vi "Array for Graph Sub VI.vi"(10 "Array in":dbl[][](array[numeric]), 11 "data":dbl[](array[numeric])) -> (2 "Cluster":cluster{dbl[], dbl[]}, 3 "Array out":dbl[][](array[numeric]))   [LabVIEW 2011]
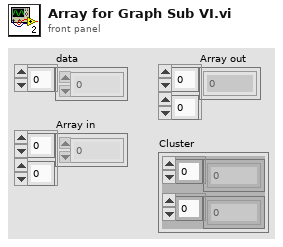
[diagram p1: front panel]
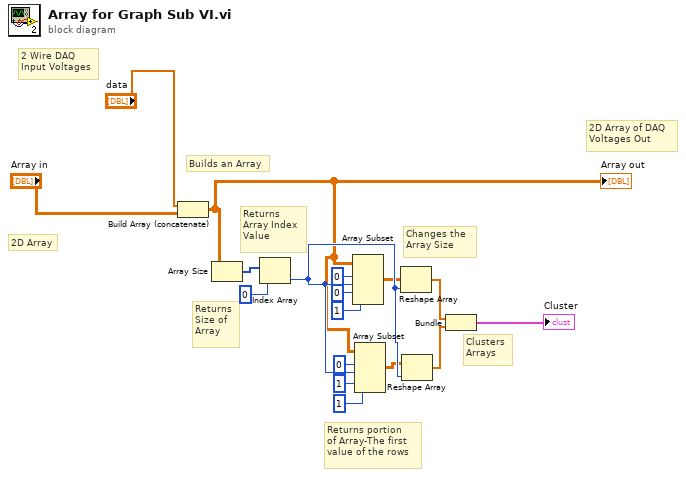
[diagram p0: block diagram]
diagram:
  # "Clusters \nArrays"
  # "Changes the \nArray Size"
  # "Returns portion \nof Array-The first \nvalue of the rows"
  # "Returns \nArray Index \nValue"
  # "Returns \nSize of \nArray"
  # "Builds an Array"
  # "2D Array of DAQ\nVoltages Out"
  # "2 Wire DAQ\nInput Voltages"
  # "2D Array"
  n1 = Build Array (concatenate)("data", "Array in") -> (w5:dbl[][])
  "Array out" <- w5
  n2 = Array Size(array=w5) -> (size(s)=w3:i32[])
  n3 = Index Array(array=w3, index=0) -> (element=w8:i32)
  n4 = Array Subset(array=w5, index (row)=0 ("index"), length (row)=w8, index (col)=0 ("index"), length (col)=1 ("length")) -> (w6:dbl[][])
  n5 = Array Subset(array=w5, index (row)=0 ("index"), length (row)=w8, index (col)=1 ("index"), length (col)=1 ("length")) -> (w7:dbl[][])
  n6 = Reshape Array(w6, w8) -> (w10:dbl[])
  n7 = Reshape Array(w7, w8) -> (w9:dbl[])
  n8 = Bundle(w10, w9) -> (→"Cluster":cluster{dbl[], dbl[]})  [unwired: 1 in]
